vi "Write Coils_Cached.vi"(8 "error in (no error)":errorcluster, 9 "Values":bool[](array[boolean]), 10 "Modbus Address":u16, 11 "MB PLC in":refnum<class "MB PLC Client.lvclass">) -> (0 "error out":errorcluster, 3 "MB PLC out":refnum<class "MB PLC Client.lvclass">)   [LabVIEW 2018, in "MB PLC Client.lvlib" / "MB PLC Client.lvclass"]
uses:
  MB PLC Client.lvclass
  MB PLC Client.lvclass/MB PLC Client.ctl
  Data/MB Data Block.lvclass
  <vilib>/Plasmionique/MB Master/MB Master.lvlib
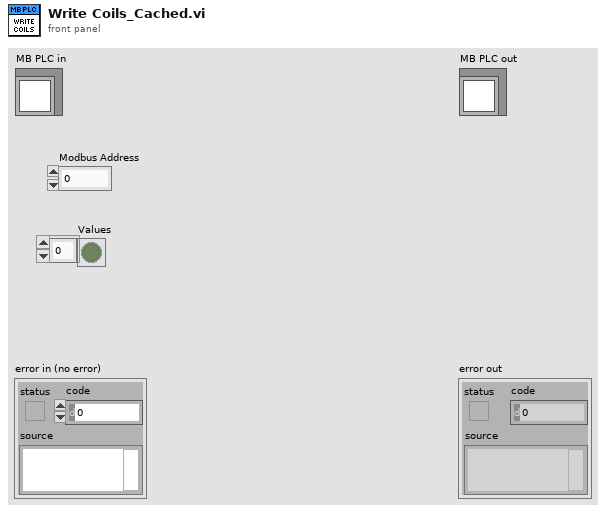
[diagram p1: front panel]
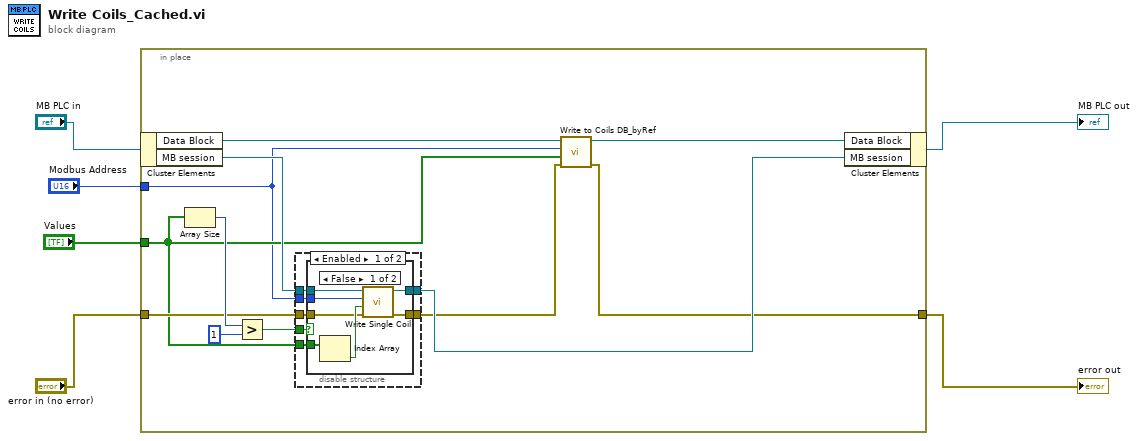
[diagram p0: block diagram]
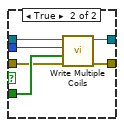
[diagram p2: hidden frame]
diagram:
  n1 = in-place {
    in-place-border: "Modbus Address" -> [w7]
    in-place-border: "Values" -> [w8]
    in-place-border: "error in (no error)" -> [w16]
    in-place-border: [w9] -> w1
    n2 = in-place-cluster #1("MB PLC in") -> ("Data Block"=w12:refnum<data-value>, "MB session"=w15:refnum<class "MB_Master.lvclass">)
    n3 = Array Size(array=w8) -> (size(s)=w18:i32)
    n4 = Greater?(x=w18, y=1) -> (0:w13:bool)
    n5 = disable-structure shown="Enabled" {
      disable-tunnel: [w25 w39] -> w10
      disable-tunnel: w16 -> [w24 w39]
      disable-tunnel: w15 -> [w23 w40]
      disable-tunnel: [w22 w40] -> w14
      disable-tunnel: w7 -> [w21 _]
      disable-tunnel: w8 -> [w20 _]
      disable-tunnel: w13 -> [w19 _]
      frame Enabled {
        n6 = case shown="False" w19 {
          tunnel: [w27 w33] -> w25
          tunnel: w24 -> [w28 w35]
          tunnel: w23 -> [w31 w38]
          tunnel: [w26 w34] -> w22
          tunnel: w21 -> [w30 w37]
          tunnel: w20 -> [w32 w36]
          frame False {
            n7 = Index Array(array=w32) -> (element=w29:bool)  [unwired: 1 in]
            n8 = call <vilib>:"Write Single Coil.vi"("error in (no error)"=w28, "value"=w29, "address"=w30, "MB session in"=w31) -> ("error out"=w27:errorcluster, "MB session out"=w26:refnum<class "MB_Master.lvclass">)  [unwired: 6 in]
          }
          frame True {
            n9 = call <vilib>:"Write Multiple Coils.vi"("error in (no error)"=w35, "values"=w36, "starting address"=w37, "MB session in"=w38) -> ("error out"=w33:errorcluster, "MB session out"=w34:refnum<class "MB_Master.lvclass">)  [unwired: 6 in]
          }
        }
      }
      frame Disabled {
      }
    }
    n10 = call "Write to Coils DB_byRef.vi"("error in (no error)"=w10, "Values"=w8, "Modbus Address"=w7, "Cache Ref in"=w12) -> ("error out"=w9:errorcluster, "Cache Ref out"=w11:refnum<data-value>)  [unwired: 6 in]
    n11 = in-place-cluster #1("Data Block"=w11, "MB session"=w14) -> (→"MB PLC out":refnum<class "MB PLC Client.lvclass">)
  }
  "error out" <- w1
